vi "error_window.vi"(7 "calling_vi":refnum<vi>, 8 "error in (no error)":errorcluster, 11 "configuration":T3) -> (0 "error out":errorcluster, 3 "dialog_selection":T4)   [LabVIEW 2015, in "lv-dialog-interfaces.lvlib"]
uses:
  lv-dialog-interfaces.lvlib
  <userlib>/antonio-alexander/lv-dialog/api/v1/public/_controls/selection.ctl
  <vilib>/Utility/error.llb/DialogTypeEnum.ctl
  <vilib>/Utility/error.llb/TagReturnType.ctl
  private/_controls/hmi_references.ctl
  private/_controls/configuration.ctl
  private/_controls/dialog_type.ctl
  <vilib>/event_ctls.llb/eventvkey.ctl
  <userlib>/antonio-alexander/lv-dialog/api/v1/v1.lvlib
panel:
  in  "Search ni.com":bool
  in  "truncated message":string="(source truncated)"
  in  "truncated & CH message":string="(source truncated; see Context Help window)"
  out "Source of Error":string
  out "scrollbar text":string
  out "?":bool=TRUE
  in  "stop":bool
  in  "continue":bool
  in  "Test for size":string
  out "text":string
  out "stop event propagated":bool
  in  "continue":bool
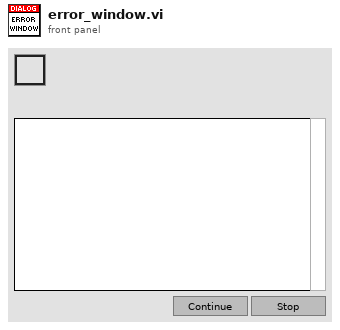
[diagram p1: front panel]
types:
  T1 = typedef "DialogTypeEnum.ctl" = enum16{"no dialog", "OK message", "continue or stop message", "auto error handling dialog", "OK message + warnings", "continue/stop + warnings"}
  T2 = typedef "TagReturnType.ctl" = enum16{"No Tag", "<err>", "<append>"}
  T3 = cluster{"Show Link":bool, "code":i32, "Length":i32[], "Start":i32[], "Source":string, "Details":string, "dialog type":T1, "Error or Warning":bool, "contname":string, "stopname":string, "okname":string, "Tag Found?":T2}
  T4 = typedef "lv-dialog.lvlib/v1.lvlib/selection.ctl" = enum16{"null", "panel_closed", "button_1", "button_2", "button_3", "cancelled"}
  T5 = typedef "lv-dialog-interfaces.lvlib/dialog_type.ctl" = enum16{"null", "one_button", "two_button", "three_button", "confirmation", "busy_wait", "error", "busy_wait_embed", "combo_box", "data_entry_string", "data_entry_numeric"}
  T6 = typedef "lv-dialog-interfaces.lvlib/configuration.ctl" = cluster{"dialog_text":string, "boolean_text_1":string, "boolean_text_2":string, "boolean_text_3":string, "inner_color":u32, "outer_color":u32, "wait_s":dbl, "error_status":bool, "error_source":string, "error_details":string, "string []":string[], "custom_entry":bool, "confirmation_text":string}
  T7 = typedef "lv-dialog-interfaces.lvlib/hmi_references.ctl" = cluster{"vi_reference":refnum<vi>, "caller":refnum<vi>, "dialog":refnum<vi>, "button_1":refnum<vi>, "button_2":refnum<vi>, "button_3":refnum<vi>, "busy":refnum<vi>, "error_glyph":refnum<vi>, "error_source":refnum<vi>, "error_text":refnum<vi>, "combo_box":refnum<vi>}
  T8 = typedef "eventvkey.ctl" = enum16{"ASCII", "Enter", "Return", "Shift", "Ctrl", "Alt", "Cmd", "Opt", "Caps", "NumLock", "Clear", "Break", "Up", "Down", "Left", "Right", "Insert", "Delete", "Home", "End", "PageUp", "PageDown", "Escape", "Help", "Pause", "ScrollLock", "F1", "F2", "F3", "F4", "F5", "F6", "F7", "F8", "F9", "F10", "F11", "F12", "F13", "F14", "F15", "F16", "F17", "F18", "F19", "F20", "F21", "F22", "F23", "F24", "Play", "VolumeUp", "VolumeDown", "Mute", "Two Byte Char"}
  T9 = typedef "LVRectTypeDef.ctl" = cluster{"Left":i16, "Top":i16, "Right":i16, "Bottom":i16}
  T10 = cluster{"Control":bool, "Shift":bool, "Key":string}
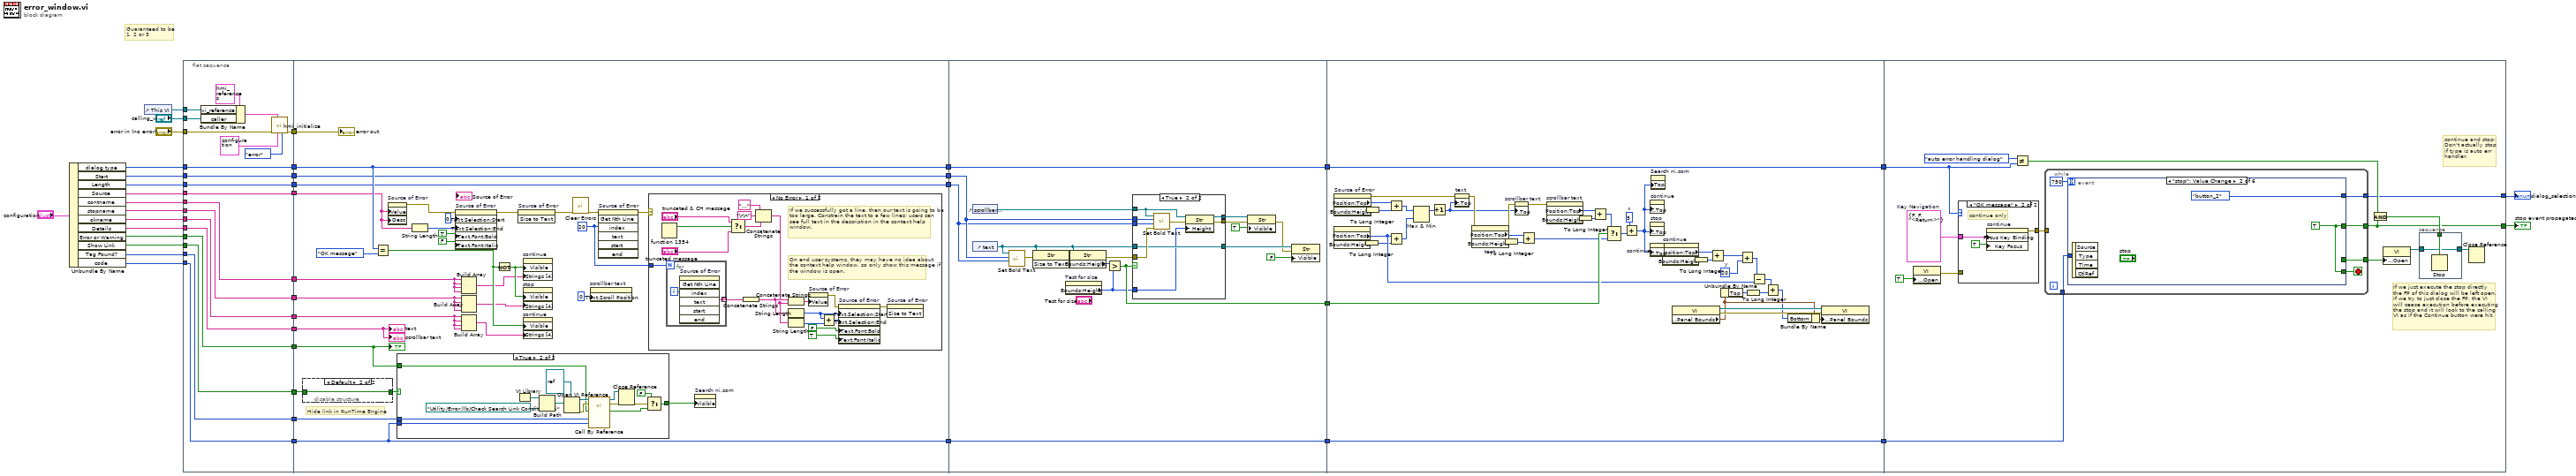
[diagram p0: block diagram]
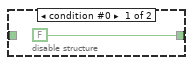
[diagram p2: hidden frame]
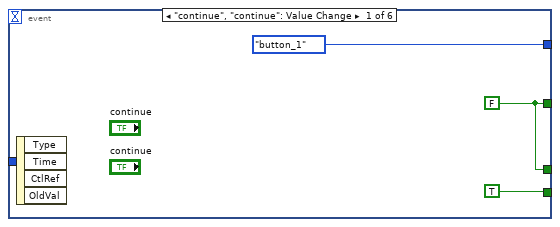
[diagram p6: hidden frame]
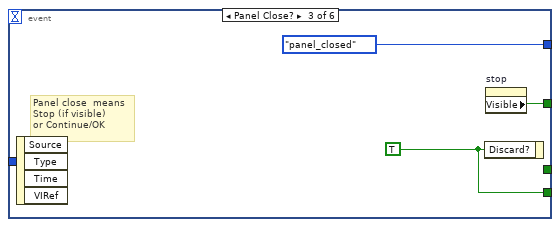
[diagram p7: hidden frame]
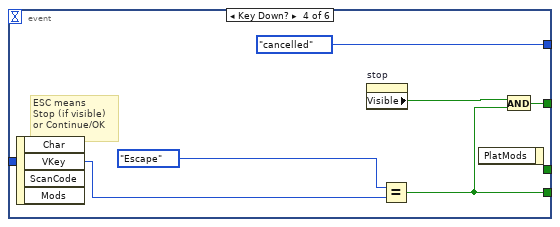
[diagram p8: hidden frame]
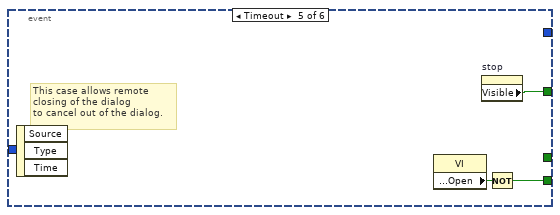
[diagram p9: hidden frame]
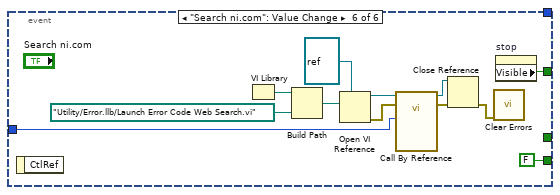
[diagram p10: hidden frame]
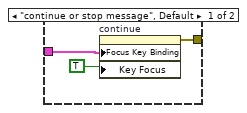
[diagram p11: hidden frame]
diagram:
  # "Guaranteed to be\n1, 2 or 3"
  n1 = Unbundle By Name("configuration") -> ("dialog type"=w13:T1, "Start"=w2:i32[], "Length"=w12:i32[], "Source"=w11:string, "contname"=w10:string, "stopname"=w9:string, "okname"=w8:string, "Details"=w7:string, "Error or Warning"=w6:bool, "Show Link"=w5:bool, "Tag Found?"=w4:T2, "code"=w3:i32)
  n2 = control-ref of="This VI"() -> (w30:refnum<vi>)
  n3 = flat-sequence {
    tunnel: "calling_vi" -> [w44]
    tunnel: w30 -> [w45]
    tunnel: w4 -> [w49]
    tunnel: w3 -> [w50]
    tunnel: w5 -> [w51]
    tunnel: w12 -> [w52]
    tunnel: w2 -> [w53]
    tunnel: w6 -> [w54]
    tunnel: w7 -> [w55]
    tunnel: w11 -> [w56]
    tunnel: w8 -> [w57]
    tunnel: w9 -> [w58]
    tunnel: w10 -> [w59]
    tunnel: w13 -> [w60]
    tunnel: [w60] -> w28
    tunnel: [w59] -> w27
    tunnel: [w58] -> w26
    tunnel: [w57] -> w25
    tunnel: [w56] -> w24
    tunnel: [w55] -> w23
    tunnel: [w54] -> w22
    tunnel: [w53] -> w21
    tunnel: [w52] -> w20
    tunnel: [w51] -> w19
    tunnel: [w50] -> w18
    tunnel: [w49] -> w17
    tunnel: "error in (no error)" -> [w42]
    tunnel: [w41] -> w15
    tunnel: [w75] -> w39
    tunnel: [w70] -> w35
    tunnel: [w69] -> w34
    tunnel: [w64] -> w31
    tunnel: w28 -> [w75]
    tunnel: w27 -> [w74]
    tunnel: w26 -> [w73]
    tunnel: w25 -> [w72]
    tunnel: w24 -> [w68]
    tunnel: w23 -> [w71]
    tunnel: w22 -> [w62]
    tunnel: w21 -> [w70]
    tunnel: w20 -> [w69]
    tunnel: w19 -> [w67]
    tunnel: w18 -> [w64]
    tunnel: w17 -> [w65]
    tunnel: w15 -> [w61]
    tunnel: w39 -> [w133]
    tunnel: [w133] -> w38
    tunnel: [w139] -> w37
    tunnel: w35 -> [w132]
    tunnel: w34 -> [w131]
    tunnel: [w130] -> w32
    tunnel: w31 -> [w130]
    tunnel: w38 -> [w168]
    tunnel: [w168] -> w36
    tunnel: w37 -> [w202]
    tunnel: [w161] -> w33
    tunnel: w32 -> [w161]
    tunnel: [w205] -> w40
    tunnel: w36 -> [w207]
    tunnel: w33 -> [w204]
    tunnel: [w203] -> w1
    frame #0 {
      n4 = Bundle By Name(cluster=T7 {"vi_reference"=refnum, "caller"=refnum, "dialog"=refnum, "button_1"=refnum, "button_2"=refnum, "button_3"=refnum, "busy"=refnum, "error_glyph"=refnum, "error_source"=refnum, "error_text"=refnum, "combo_box"=refnum} ("references"), "vi_reference"=w45, "caller"=w44) -> (w43:T7)
      n5 = call "hmi_initialize.vi"("dialog_type"=dialog_type."error", "configuration"=T6 {"dialog_text"="", "boolean_text_1"="", "boolean_text_2"="", "boolean_text_3"="", "inner_color"=16711680, "outer_color"=6618880, "wait_s"=nan, "error_status"=FALSE, "error_source"="", "error_details"="", "string []"=[], "custom_entry"=FALSE, "confirmation_text"=""}, "references"=w43, "error in (no error)"=w42) -> ("error out"=w41:errorcluster)  [unwired: 7 in]
    }
    frame #1 {
      w82 = u32 20 ("index")
      # "Hide link in RunTime Engine"
      n6 = disable-structure shown="Default" {
        disable-tunnel: w67 -> [_ w94]
        disable-tunnel: [FALSE ("Show Link") w94] -> w66
        frame condition #0 {
        }
        frame condition #1 (active) {
        }
      }
      n7 = Equal?(x=w75, y=DialogTypeEnum."OK message" ("dialog type")) -> (x = y?=w92:bool)
      n8 = property on="Source of Error" class="Str"("Value"=w68, "Desc"=w68) -> (error out=w81:errorcluster)  [unwired: 2 in, 1 out]
      n9 = case shown="True" w66 {
        tunnel: [_ w102] -> w63
        tunnel: w65 -> [_ w101]
        tunnel: w64 -> [_ w100]
        tunnel: w62 -> [_ w99]
        frame False {
        }
        frame True {
          n10 = VI Library() -> (path=w108:path)
          n11 = Build Path(base path=w108, name or relative path=path "Utility/Error.llb/Check Search Link Conditions.vi") -> (appended path=w109:path)
          n12 = Open VI Reference(type specifier VI Refnum (for type only)=refnum<vi> refnum, vi path=w109) -> (vi reference=w105:refnum<vi>, error out=w107:errorcluster)  [unwired: 4 in]
          n13 = call-by-ref "?"(reference=w105, error in=w107, "Error Code"=w100, "Tag Found?"=w101, "Error or Warning?"=w99) -> (reference out=w98:refnum<vi>, error out=w97:errorcluster, "Display Link?"=w104:bool)  [unwired: 8 in]
          n14 = Close Reference(reference=w98, error in (no error)=w97) -> (error out=w96:errorcluster)
          n15 = Select(t=FALSE, s=w96, f=w104) -> (s? t:f=w102:bool)
        }
      }
      n16 = String Length(string=w68) -> (length=w78:i32)
      n17 = property on="Source of Error" class="Str"(error in=w81, "Text.Selection:Start"=u32 0, "Text.Selection:End"=w78, "Text.Font:Bold"=TRUE, "Text.Font:Italic"=FALSE) -> (error out=w80:errorcluster)  [unwired: 1 in, 1 out]
      n18 = Build Array(w74, w74, w74, w74) -> (w90:string[])
      n19 = Build Array(w73, w73, w73, w73) -> (w89:string[])
      n20 = Build Array(w72, w72, w72, w72) -> (w88:string[])
      n21 = Not(x=w92) -> (.not. x?=w91:bool)
      n22 = invoke on="Source of Error" class="Str" method="Size to Text"(error in=w80) -> (error out=w85:errorcluster)  [unwired: 2 in, 2 out]
      n23 = property on="continue" class="Bool"("Visible"=w91, "Strings [4]"=w90) -> ()  [unwired: 2 in, 2 out]
      n24 = property on="stop" class="Bool"("Visible"=w91, "Strings [4]"=w89) -> ()  [unwired: 2 in, 2 out]
      n25 = property on="continue" class="Bool"("Visible"=w92, "Strings [4]"=w88) -> ()  [unwired: 2 in, 2 out]
      n26 = call <vilib>:"Clear Errors.vi"("error in (no error)"=w85) -> ("error out"=w84:errorcluster)  [unwired: 5 in, 1 out]
      n27 = property on="scrollbar text" class="Str"("Text.Scroll Position"=u32 0) -> ()  [unwired: 2 in, 2 out]
      n28 = invoke on="Source of Error" class="Str" method="Get Nth Line"(error in=w84, "index"=w82) -> (error out=w83:errorcluster)  [unwired: 5 in, 6 out]
      n29 = case shown="No Error" w83 {
        tunnel: w82 -> [w127 _]
        frame No Error {
          # "If we successfully got a line, then our text is going to be too large. Constrain the text to a few lines; users can see full text in the description in the context help window."
          # "On end user systems, they may have no idea about\nthe context help window, so only show this message if\nthe window is open."
          n30 = fn#1354() -> (1:w117:bool)  [unwired: 1 out]
          n31 = for {
            N: w127 -> [_]
            tunnel: [w128] -> w125 mode=indexing
            i -> [w129]
            n32 = invoke on="Source of Error" class="Str" method="Get Nth Line"("index"=w129) -> ("text"=w128:string)  [unwired: 6 in, 6 out]
          }
          n33 = Select(t="truncated & CH message", s=w117, f="truncated message") -> (s? t:f=w114:string)
          n34 = Concatenate Strings(w125) -> (w124:string)
          n35 = Concatenate Strings("..." ("string"), "\r\n", w114) -> (w111:string)
          n36 = Concatenate Strings(w124, w111) -> (w126:string)
          n37 = String Length(string=w124) -> (length=w119:i32)
          n38 = String Length(string=w111) -> (length=w116:i32)
          n39 = property on="Source of Error" class="Str"("Value"=w126) -> (error out=w121:errorcluster)  [unwired: 2 in, 1 out]
          n40 = Add(x=w119, y=w116) -> (x+y=w118:i32)
          n41 = property on="Source of Error" class="Str"(error in=w121, "Text.Selection:Start"=w119, "Text.Selection:End"=w118, "Text.Font:Bold"=FALSE, "Text.Font:Italic"=TRUE) -> (error out=w120:errorcluster)  [unwired: 1 in, 1 out]
          n42 = invoke on="Source of Error" class="Str" method="Size to Text"(error in=w120) -> ()  [unwired: 2 in, 3 out]
        }
        frame Error {
          # "An error at this point means that there is no line to fetch. That's good. We do not want the text getting too large."
        }
      }
      n43 = property on="Search ni.com" class="Bool"("Visible"=w63) -> ()  [unwired: 2 in, 2 out]
      "?" <- w62
      "scrollbar text" <- w71
      "text" <- w71
      "error out" <- w61
    }
    frame #2 {
      n44 = control-ref of="scrollbar text"() -> (w142:refnum<vi>)
      n45 = control-ref of="text"() -> (w134:refnum<vi>)
      n46 = call <vilib>:"Set Bold Text.vi"("Length"=w131, "Start"=w132, "text"=w134) -> ("error out"=w137:errorcluster)  [unwired: 3 in]
      n47 = invoke class="Str" method="Size to Text"(reference=w134, error in=w137) -> (error out=w138:errorcluster)  [unwired: 1 in, 2 out]
      n48 = property on="Test for size" class="Str"() -> ("Bounds:Height"=w136:u32)  [unwired: 2 in, 2 out]
      n49 = property class="Str"(reference=w134, error in=w138) -> (error out=w146:errorcluster, "Bounds:Height"=w147:u32)  [unwired: 1 out]
      n50 = Greater?(x=w147, y=w136) -> (0:w139:bool)
      n51 = case shown="True" w139 {
        tunnel: w146 -> [w150 w159]
        tunnel: w132 -> [_ w158]
        tunnel: w131 -> [_ w157]
        tunnel: [w150 w154] -> w135
        tunnel: w134 -> [w149 w156]
        tunnel: [w149 w151] -> w144
        tunnel: [w148 w156] -> w143
        tunnel: w142 -> [w148 w152]
        tunnel: w136 -> [_ w155]
        frame False {
        }
        frame True {
          n52 = call <vilib>:"Set Bold Text.vi"("error in"=w159, "Length"=w157, "Start"=w158, "text"=w152) -> ("error out"=w153:errorcluster)  [unwired: 2 in]
          n53 = property class="Str"(reference=w152, error in=w153, "Height"=w155) -> (reference out=w151:refnum<vi>, error out=w154:errorcluster)
        }
      }
      n54 = property class="Str"(reference=w144, error in=w135, "Visible"=TRUE ("Defer Panel Updates")) -> (error out=w140:errorcluster)  [unwired: 1 out]
      n55 = property class="Str"(reference=w143, error in=w140, "Visible"=FALSE ("Defer Panel Updates")) -> ()  [unwired: 2 out]
    }
    frame #3 {
      w189 = 20  # y
      w194 = 5  # x
      n56 = property class="Bool"() -> ("Position:Top"=w184:i32, "Bounds:Height"=w199:u32)  [unwired: 2 in, 2 out]
      n57 = property on="Source of Error" class="Str"() -> (error out=w169:errorcluster, "Position:Top"=w171:i32, "Bounds:Height"=w170:u32)  [unwired: 2 in, 1 out]
      n58 = To Long Integer(number=w199) -> (32bit integer=w167:i32)
      n59 = To Long Integer(number=w170) -> (32bit integer=w166:i32)
      n60 = Add(x=w171, y=w166) -> (x+y=w201:i32)
      n61 = Add(x=w184, y=w167) -> (x+y=w200:i32)
      n62 = Max & Min(x=w201, y=w200) -> (max(x,y)=w198:i32)  [unwired: 1 out]
      n63 = Increment(x=w198) -> (x+1=w177:i32)
      n64 = property on="text" class="Str"(error in=w169, "Position:Top"=w177) -> (error out=w179:errorcluster)  [unwired: 1 in, 1 out]
      n65 = property on="text" class="Str"(error in=w179) -> (error out=w178:errorcluster, "Position:Top"=w176:i32, "Bounds:Height"=w175:u32)  [unwired: 1 in, 1 out]
      n66 = To Long Integer(number=w175) -> (32bit integer=w165:i32)
      n67 = property on="scrollbar text" class="Str"(error in=w178, "Position:Top"=w177) -> (error out=w197:errorcluster)  [unwired: 1 in, 1 out]
      n68 = Add(x=w176, y=w165) -> (x+y=w173:i32)
      n69 = property on="scrollbar text" class="Str"(error in=w197) -> ("Position:Top"=w196:i32, "Bounds:Height"=w195:u32)  [unwired: 1 in, 2 out]
      n70 = To Long Integer(number=w195) -> (32bit integer=w164:i32)
      n71 = Add(x=w196, y=w164) -> (x+y=w174:i32)
      n72 = Select(t=w174, s=w202, f=w173) -> (s? t:f=w172:i32)
      n73 = Add(x=w194, y=w172) -> (x+y=w160:i32)
      n74 = property on="continue" class="Bool"("Position:Top"=w160) -> ()  [unwired: 2 in, 2 out]
      n75 = property on="stop" class="Bool"("Position:Top"=w160) -> ()  [unwired: 2 in, 2 out]
      n76 = property on="continue" class="Bool"("Position:Top"=w160) -> (error out=w193:errorcluster)  [unwired: 2 in, 1 out]
      n77 = property on="Search ni.com" class="Bool"("Top"=w160) -> ()  [unwired: 2 in, 2 out]
      n78 = property on="continue" class="Bool"(error in=w193) -> ("Position:Top"=w191:i32, "Bounds:Height"=w192:u32)  [unwired: 1 in, 2 out]
      n79 = property class="VI"() -> (reference out=w186:refnum<vi>, error out=w187:errorcluster, "Front Panel Window:Panel Bounds"=w183:T9)  [unwired: 2 in]
      n80 = To Long Integer(number=w192) -> (32bit integer=w163:i32)
      n81 = Add(x=w191, y=w163) -> (x+y=w190:i32)
      n82 = Unbundle By Name(w183) -> ("Top"=w181:i16)
      n83 = Add(x=w190, y=w189) -> (x+y=w185:i32)
      n84 = To Long Integer(number=w181) -> (32bit integer=w162:i32)
      n85 = Subtract(x=w185, y=w184) -> (x-y=w182:i32)
      n86 = Add(x=w182, y=w162) -> (x+y=w180:i32)
      n87 = Bundle By Name(cluster=w183, "Bottom"=w180) -> (w188:T9)
      n88 = property class="VI"(reference=w186, error in=w187, "Front Panel Window:Panel Bounds"=w188) -> ()  [unwired: 2 out]
    }
    frame #4 {
      w216 = T10 {"Control"=FALSE, "Shift"=FALSE, "Key"="<Return>"}  # Key Navigation
      # "If we just execute the stop directly\nthe FP of this dialog will be left open.\nIf we try to just close the FP, the VI\nwill cease execution before executing\nthe stop and it will look to the calling\nVI as if the Continue button were hit."
      # "continue and stop;\nDon't actually stop\nif type is auto err\nhandler."
      n89 = property class="VI"("Front Panel Window:Open"=TRUE) -> (error out=w215:errorcluster)  [unwired: 2 in, 1 out]
      n90 = case shown="\"OK message\"" w207 {
        tunnel: w216 -> [w256 w259]
        tunnel: w215 -> [_ _]
        tunnel: [w254 w257] -> w213
        frame "continue or stop message", Default {
          n91 = property on="continue" class="Bool"("Focus Key Binding"=w256, "Key Focus"=TRUE) -> (error out=w254:errorcluster)  [unwired: 2 in, 1 out]
        }
        frame "OK message" {
          # "continue only"
          n92 = property on="continue" class="Bool"("Focus Key Binding"=w259, "Key Focus"=TRUE) -> (error out=w257:errorcluster)  [unwired: 2 in, 1 out]
        }
      }
      n93 = Not Equal?(x=DialogTypeEnum."auto error handling dialog" ("dialog type"), y=w207) -> (x != y?=w212:bool)
      n94 = while {
        tunnel: w213 -> [_]
        tunnel: [w223] -> w205
        tunnel: [w222] -> w206
        tunnel: w204 -> [w220]
        tunnel: [w219] -> w203
        stop <- w224 stop-if-true
        n95 = event shown="[1] \"stop\": Value Change" {
          selector: _ -> [_ _ _ _ _ _]
          dyn-events: _ -> [_ _ _ _ _ _]
          timeout: 750 -> [_ _ _ _ _ _]
          tunnel: [TRUE ("Stop") w228 w232 w234 w239 FALSE ("Discard?")] -> w224
          tunnel: [w227 w228 w231 w237 w241 w253] -> w223
          tunnel: [w227 _ _ _ _ _] -> w222
          tunnel: w220 -> [_ _ _ _ _ w246]
          tunnel: [selection."button_1" ("dialog_selection") selection."button_2" ("dialog_selection") selection."panel_closed" ("dialog_selection") selection."cancelled" ("dialog_selection") _ _] -> w219
          event "continue", "continue": Value Change {
            w227 = FALSE ("Stop")
            n96 = event-data() -> ()  [unwired: 1 in, 4 out]
          }
          event "stop": Value Change {
            w228 = TRUE
            n97 = event-data() -> ()  [unwired: 1 in, 4 out]
          }
          event Panel Close? {
            w232 = TRUE ("Discard?")
            # "Panel close  means\nStop (if visible)\nor Continue/OK"
            n98 = event-data() -> ()  [unwired: 1 in, 4 out]
            n99 = event-data("Discard?"=w232) -> ()  [unwired: 1 in, 1 out]
            n100 = property on="stop" class="Bool"() -> ("Visible"=w231:bool)  [unwired: 2 in, 2 out]
          }
          event Key Down? {
            # "ESC means\nStop (if visible)\nor Continue/OK"
            n101 = event-data() -> ("VKey"=w236:T8)  [unwired: 1 in, 3 out]
            n102 = property on="stop" class="Bool"() -> ("Visible"=w238:bool)  [unwired: 2 in, 2 out]
            n103 = Equal?(x=eventvkey."Escape", y=w236) -> (x = y?=w234:bool)
            n104 = event-data() -> ()  [unwired: 2 in, 1 out]
            n105 = And(x=w238, y=w234) -> (x .and. y?=w237:bool)
          }
          event Timeout {
            # "This case allows remote\nclosing of the dialog\nto cancel out of the dialog."
            n106 = event-data() -> ()  [unwired: 1 in, 3 out]
            n107 = property class="VI"() -> ("Front Panel Window:Open"=w240:bool)  [unwired: 2 in, 2 out]
            n108 = property on="stop" class="Bool"() -> ("Visible"=w241:bool)  [unwired: 2 in, 2 out]
            n109 = Not(x=w240) -> (.not. x?=w239:bool)
          }
          event "Search ni.com": Value Change {
            n110 = event-data() -> ()  [unwired: 1 in, 1 out]
            n111 = VI Library() -> (path=w248:path)
            n112 = Build Path(base path=w248, name or relative path=path "Utility/Error.llb/Launch Error Code Web Search.vi") -> (appended path=w247:path)
            n113 = Open VI Reference(type specifier VI Refnum (for type only)=refnum<vi> refnum, vi path=w247) -> (vi reference=w251:refnum<vi>, error out=w249:errorcluster)  [unwired: 4 in]
            n114 = call-by-ref "?"(reference=w251, error in=w249, "Code"=w246) -> (reference out=w245:refnum<vi>, error out=w244:errorcluster)  [unwired: 11 in]
            n115 = Close Reference(reference=w245, error in (no error)=w244) -> (error out=w243:errorcluster)
            n116 = call <vilib>:"Clear Errors.vi"("error in (no error)"=w243) -> ()  [unwired: 5 in, 2 out]
            n117 = property on="stop" class="Bool"() -> ("Visible"=w253:bool)  [unwired: 2 in, 2 out]
          }
        }
      }
      n118 = And(x=w212, y=w205) -> (x .and. y?=w211:bool)
      n119 = property class="VI"("Front Panel Window:Open"=w206) -> (reference out=w209:refnum<vi>)  [unwired: 2 in, 1 out]
      n120 = stacked-sequence {
        tunnel: w209 -> [w217]
        tunnel: w211 -> [w218]
        tunnel: [w217] -> w210
        frame #0 {
          n121 = Stop(stop? (T)=w218) -> ()
        }
      }
      n122 = Close Reference(reference=w210) -> ()  [unwired: 1 in, 1 out]
    }
  }
  "stop event propagated" <- w40
  "dialog_selection" <- w1
